vi "ABR3-Threshold Warning Dialog.vi"(0 "Result":T1, 2 "Parent VI":refnum<vi>) -> ()   [LabVIEW 2020]
uses:
  ABR3-Threshold Estimation Result.ctl
panel:
  in  "tabs":enum32{"supra", "noisy"}(tab)
  in  "OK Button":bool
  # "All of the ABR responses are suprathreshold. \n\nConsider testing using lower stimulus levels."
  # "The ABR data are noisy. Visually confirm the suggested threshold\n\nConsider testing using higher stimulus levels."
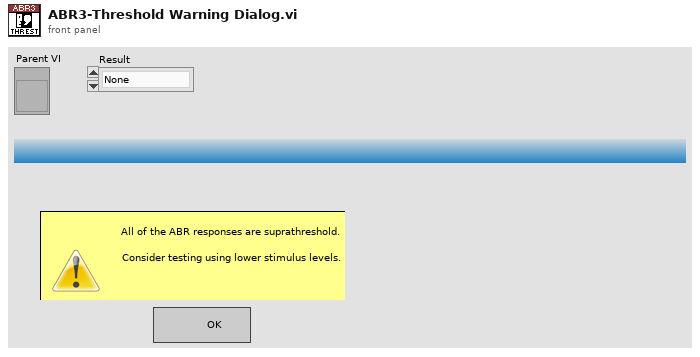
[diagram p1: front panel]
types:
  T1 = typedef "ABR3-Threshold Estimation Result.ctl" = enum16{"None", "Power", "Sigmoid", "Power (noisy)", "Suprathreshold", "Invalid"}
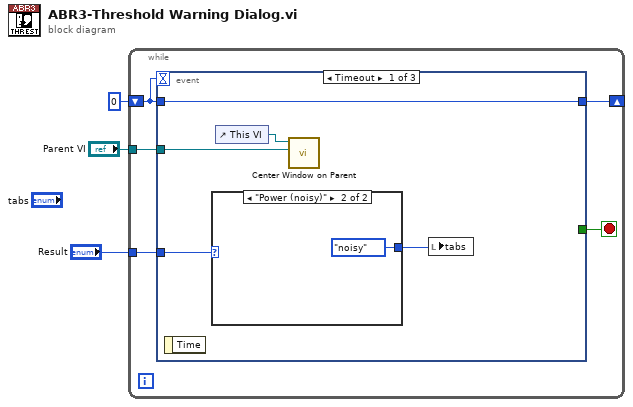
[diagram p0: block diagram]
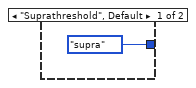
[diagram p2: hidden frame]
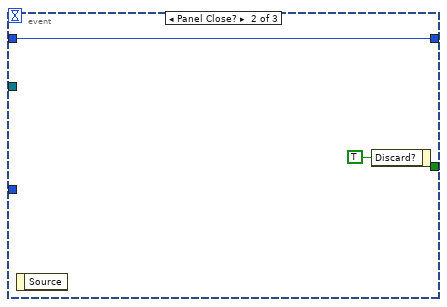
[diagram p3: hidden frame]
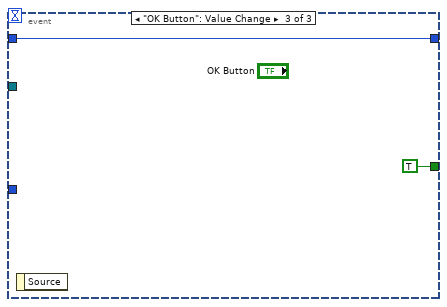
[diagram p4: hidden frame]
diagram:
  n1 = while {
    shift-right: [w7] -> _
    shift-left: 0 -> [w8]
    tunnel: "Parent VI" -> [w5]
    tunnel: "Result" -> [w4]
    stop <- w6 stop-if-true
    n2 = event shown="[0] Timeout" {
      selector: _ -> [_ _ _]
      dyn-events: _ -> [_ _ _]
      timeout: w8 -> [_ _ _]
      tunnel: w8 -> [w13 w16 w19]
      tunnel: [w13 w16 w19] -> w7
      tunnel: [_ _ TRUE] -> w6
      tunnel: w5 -> [w12 _ _]
      tunnel: w4 -> [w10 _ _]
      event Timeout {
        n3 = event-data() -> ()  [unwired: 1 in, 1 out]
        n4 = case shown="\"Power (noisy)\"" w10 {
          tunnel: [enum32{"supra", "noisy"}."supra" ("tabs") enum32{"supra", "noisy"}."noisy" ("tabs")] -> w9
          frame "Suprathreshold", Default {
          }
          frame "Power (noisy)" {
          }
        }
        n5 = control-ref of="This VI"() -> (w11:refnum<vi>)
        n6 = call "Center Window on Parent.vi"("Parent VI"=w12, "VI in"=w11) -> ()  [unwired: 8 in, 2 out]
        n7 = local write "tabs"(w9) -> ()
      }
      event Panel Close? {
        n8 = event-data() -> ()  [unwired: 1 in, 1 out]
        n9 = event-data("Discard?"=TRUE) -> ()  [unwired: 1 in, 1 out]
      }
      event "OK Button": Value Change {
        n10 = event-data() -> ()  [unwired: 1 in, 1 out]
      }
    }
  }
